vi "single_device_dserver_template.vi"(1 "?":bool, 2 "Instance Name":string, 3 "Executable Name":string) -> (0 "Device List":string[](array[string]))   [LabVIEW 2014]
uses:
  vis/tango_vi.llb/tango.lvlib
  vis/tango_vi.llb/_TangoState_t.ctl
  vis/tango_vi.llb/_DServerSetStringScalarAttributeValue.vi
  vis/tango_vi.llb/_DServerSetStateScalarAttributeValue.vi
  examples.llb/sinewavercontrols.vi
  vis/tango_vi.llb/_DServerSetDoubleScalarAttributeValue.vi
  vis/tango_vi.llb/_DServerRequestDataToDoubleScalar.vi
  vis/tango_vi.llb/_DServerClientRequestType.ctl
  vis/tango_vi.llb/_DataType.ctl
  vis/tango_vi.llb/_GenericDataBuffer.ctl
  vis/tango_vi.llb/_DServerClientRequestData.ctl
  vis/tango_vi.llb/_DServerClientRequest.ctl
panel:
  out "Client Request":T1={"Request Id"=0, "Source Id"=0, "Request Type"=enum."UNKNOWN_REQUEST", "Device Class Name"="unspecified_class_name", "Device Name"="unspecified/device/name", "Cmd or Attr Name"="unspecified_cmd_or_attr_name", "Client Request Data"={"write attribute value"={"dimx"=0, "dimy"=0, "data"=[], "data_type"=enum."UNKNOWN_DATA_TYPE"}, "exec. command argin"={"num data"=[], "str data"=[]}}}
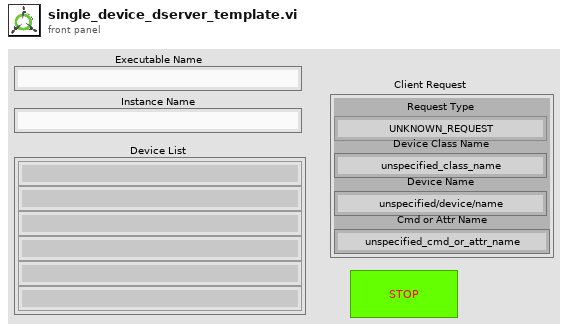
[diagram p1: front panel]
types:
  T1 = typedef "tango.lvlib/_DServerClientRequest.ctl" = cluster{"Request Id":u32, "Source Id":u32, "Request Type":T2, "Device Class Name":string, "Device Name":string, "Cmd or Attr Name":string, "Client Request Data":T3}
  T2 = typedef "tango.lvlib/_DServerClientRequestType.ctl" = enum16{"EXEC_CMD", "READ_ATTR", "WRITE_ATTR", "UNKNOWN_REQUEST"}
  T3 = typedef "tango.lvlib/_DServerClientRequestData.ctl" = cluster{"write attribute value":T4, "exec. command argin":cluster{"num data":u8[], "str data":string[]}}
  T4 = typedef "tango.lvlib/_GenericDataBuffer.ctl" = cluster{"dimx":u32, "dimy":u32, "data":u8[], "data_type":T5}
  T5 = typedef "tango.lvlib/_DataType.ctl" = enum16{"STATE_SCA", "STATE_SPE", "STATE_IMG", "STRING_SCA", "STRING_SPE", "STRING_IMG", "BOOL_SCA", "BOOL_SPE", "BOOL_IMG", "UCHAR_SCA", "UCHAR_SPE", "UCHAR_IMG", "SHORT_SCA", "SHORT_SPE", "SHORT_IMG", "USHORT_SCA", "USHORT_SPE", "USHORT_IMG", "LONG_SCA", "LONG_SPE", "LONG_IMG", "ULONG_SCA", "ULONG_SPE", "ULONG_IMG", "LONG64_SCA", "LONG64_SPE", "LONG64_IMG", "ULONG64_SCA", "ULONG64_SPE", "ULONG64_IMG", "FLOAT_SCA", "FLOAT_SPE", "FLOAT_IMG", "DOUBLE_SCA", "DOUBLE_SPE", "DOUBLE_IMG", "SCA_ENCODED", "SPE_ENCODED", "IMG_ENCODED", "UNKNOWN_DATA_TYPE"}
  T6 = typedef "_DServerEvent.ctl" = cluster{"event registration refnum":refnum<event-registration>, "user event out":refnum<user-event>}
  T7 = typedef "tango.lvlib/_TangoState_t.ctl" = enum32{"ON", "OFF", "CLOSE", "OPEN", "INSERT", "EXTRACT", "MOVING", "STANDBY", "FAULT", "INIT", "RUNNING", "ALARM", "DISABLE", "UNKNOWN"}
  T8 = typedef "_DServerClientRequest.ctl" = cluster{"Request Id":u32, "Source Id":u32, "Request Type":T9, "Device Class Name":string, "Device Name":string, "Cmd or Attr Name":string, "Client Request Data":T10}
  T9 = typedef "_DServerClientRequestType.ctl" = enum16{"EXEC_CMD", "READ_ATTR", "WRITE_ATTR", "UNKNOWN_REQUEST"}
  T10 = typedef "_DServerClientRequestData.ctl" = cluster{"write attribute value":T11, "exec. command argin":cluster{"num data":u8[], "str data":string[]}}
  T11 = typedef "_GenericDataBuffer.ctl" = cluster{"dimx":u32, "dimy":u32, "data":u8[], "data_type":T5}
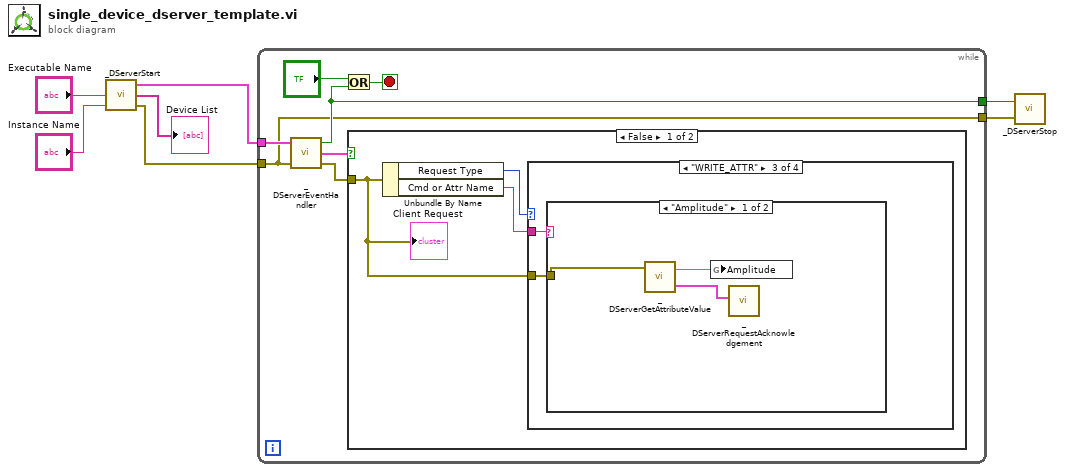
[diagram p0: block diagram]
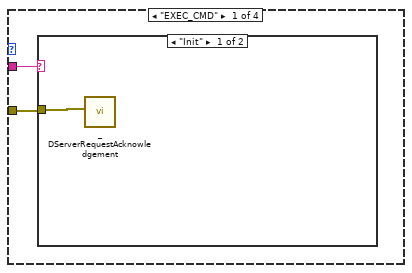
[diagram p2: hidden frame]
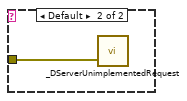
[diagram p3: hidden frame]
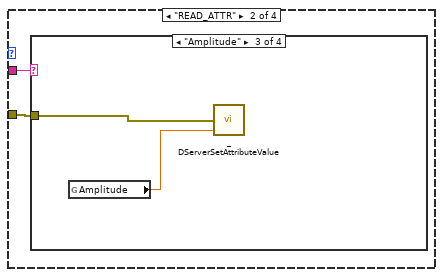
[diagram p4: hidden frame]
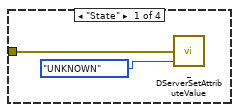
[diagram p5: hidden frame]
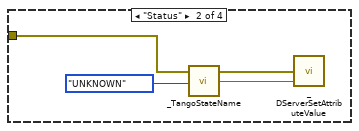
[diagram p6: hidden frame]
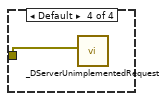
[diagram p7: hidden frame]
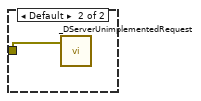
[diagram p8: hidden frame]
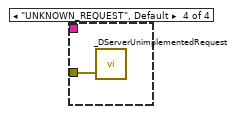
[diagram p9: hidden frame]
diagram:
  n1 = call "_DServerStart.vi"("error in"="Instance Name", "instance name"="Executable Name") -> ("error out"=w7:errorcluster, "device_list"=→"Device List":string[], "dserver evt."=w1:T6)  [unwired: 1 in]
  n2 = while {
    tunnel: [w10] -> w5
    tunnel: w7 -> [w9]
    tunnel: w1 -> [w13]
    tunnel: [w9] -> w4
    stop <- w8 stop-if-true
    n3 = call "_DServerEventHandler.vi"("error in"=w9, "timeout"=w13) -> ("error out"=w11:errorcluster, "client request"=w14:T8, "timeout"=w10:bool)  [unwired: 1 in]
    n4 = Or(x="?", y=w10) -> (x .or. y?=w8:bool)
    n5 = case shown="False" w14 {
      tunnel: w11 -> [w17 _]
      frame False {
        n6 = Unbundle By Name(w17) -> ("Request Type"=w15:T2, "Cmd or Attr Name"=w16:string)
        n7 = case shown="\"WRITE_ATTR\"" w15 {
          tunnel: w16 -> [w18 w23 w32 _]
          tunnel: w17 -> [w19 w22 w33 w38]
          frame "EXEC_CMD" {
            n8 = case shown="\"Init\"" w18 {
              tunnel: w19 -> [w20 w21]
              frame "Init" {
                n9 = call "_DServerRequestAcknowledgement.vi"("client request"=w20) -> ()  [unwired: 3 in, 1 out]
              }
              frame Default {
                n10 = call "_DServerUnimplementedRequest.vi"("client request"=w21) -> ()  [unwired: 1 in, 1 out]
              }
            }
          }
          frame "READ_ATTR" {
            n11 = case shown="\"Amplitude\"" w23 {
              tunnel: w22 -> [w24 w27 w30 w31]
              frame "State" {
                n12 = call-poly "_DServerSetAttributeValue.vi"("value"=_TangoState_t."UNKNOWN" ("Tango Device State"), "client request"=w24) -> ()  [unwired: 1 in, 1 out]
              }
              frame "Status" {
                n13 = call "_TangoStateName.vi"("State"=_TangoState_t."UNKNOWN" ("Tango Device State")) -> ("State Name"=w28:string)
                n14 = call-poly "_DServerSetAttributeValue.vi"("value"=w28, "client request"=w27) -> ()  [unwired: 1 in, 1 out]
              }
              frame "Amplitude" {
                n15 = global read "sinewavercontrols.vi" "Amplitude"() -> (w29:dbl)
                n16 = call-poly "_DServerSetAttributeValue.vi"("value"=w29, "client request"=w30) -> ()  [unwired: 1 in, 1 out]
              }
              frame Default {
                n17 = call "_DServerUnimplementedRequest.vi"("client request"=w31) -> ()  [unwired: 1 in, 1 out]
              }
            }
          }
          frame "WRITE_ATTR" {
            n18 = case shown="\"Amplitude\"" w32 {
              tunnel: w33 -> [w36 w37]
              frame "Amplitude" {
                n19 = call-poly "_DServerGetAttributeValue.vi"("client request"=w36) -> ("attribute value"=w35:dbl, "client request"=w34:T8)
                n20 = global write "sinewavercontrols.vi" "Amplitude"(w35) -> ()
                n21 = call "_DServerRequestAcknowledgement.vi"("client request"=w34) -> ()  [unwired: 3 in, 1 out]
              }
              frame Default {
                n22 = call "_DServerUnimplementedRequest.vi"("client request"=w37) -> ()  [unwired: 1 in, 1 out]
              }
            }
          }
          frame "UNKNOWN_REQUEST", Default {
            n23 = call "_DServerUnimplementedRequest.vi"("client request"=w38) -> ()  [unwired: 1 in, 1 out]
          }
        }
        "Client Request" <- w17
      }
      frame True {
      }
    }
  }
  n24 = call "_DServerStop.vi"("dserver evt."=w4, "error in"=w5) -> ()  [unwired: 1 out]
